vi "practica9.vi"() -> ()   [LabVIEW 2016]
panel:
  in  "file path (use dialog) 2":path
  out "Waveform derecho 2":dbl[](graph)
  out "Waveform izquierdo":dbl[](graph)
  in  "file path (use dialog)":path
  out "Angulo":dbl
  out "Plano de trabajo":picture
  in  "Reset":bool
  in  "stop":bool
  out "Motor Izquierda":dbl(slide) scale=-100.0..100.0
  out "Motor Derecha":dbl(slide) scale=-100.0..100.0
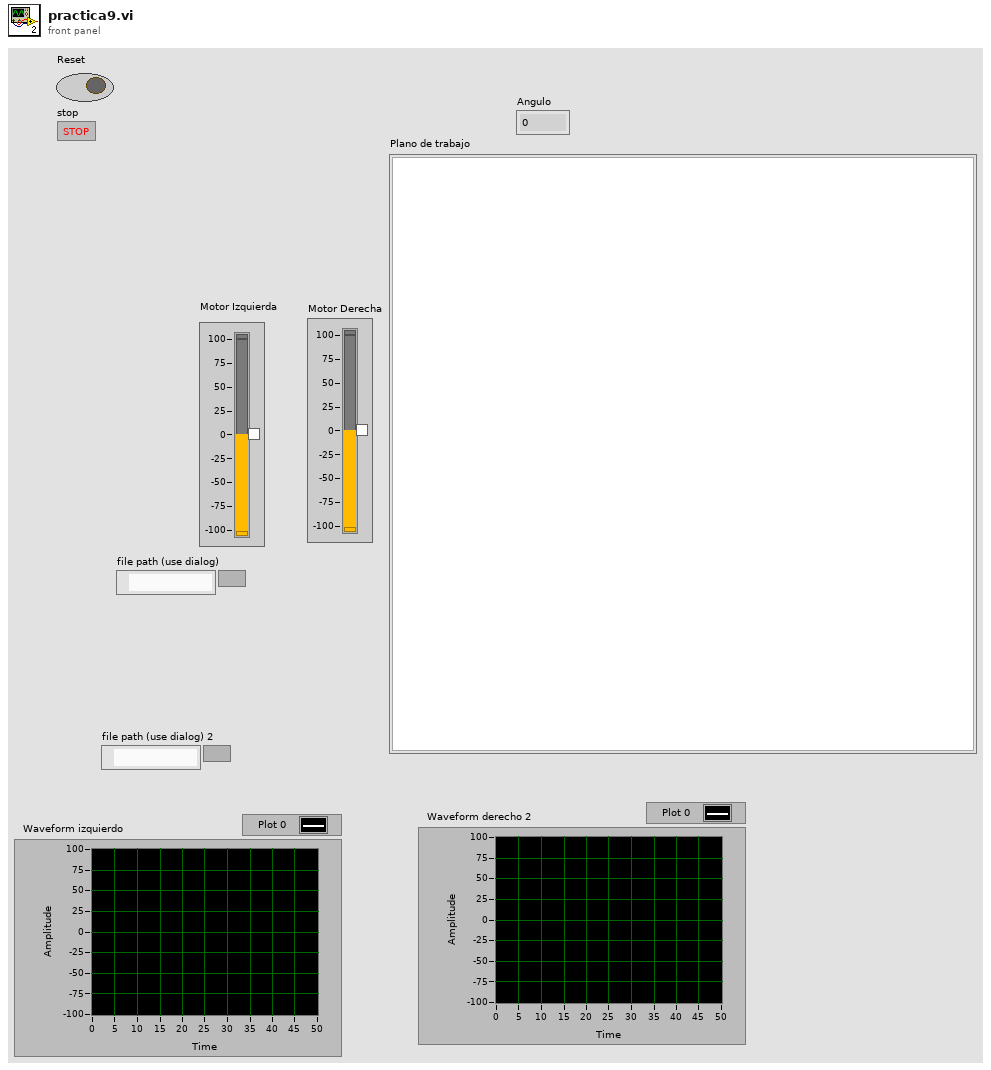
[diagram p1: front panel]
types:
  T1 = enum16{"open", "replace", "create", "open or create", "replace or create", "replace or create with confirmation"}
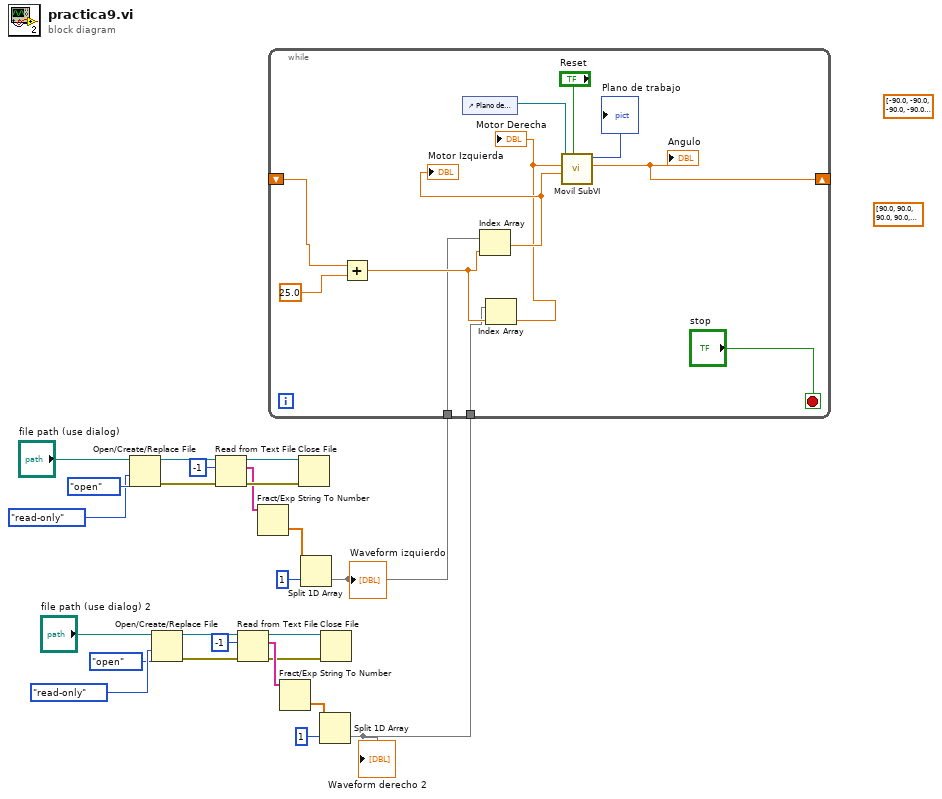
[diagram p0: block diagram]
diagram:
  (unwired) dbl[] [90.0, 90.0, 90.0, 90.0, 90.0, 90.0, 90.0, 90.0, 90.0, 90.0, 90.0, 82.0, 74.0, 66.0, 58.0, 50.0, 50.0, 50.0, 50.0, 50.0, 50.0, 33.3333333333333, 21.4285714285714, 12.5, 5.55555555555556, 0.0, -5.55555555555556, -12.5, -21.4285714285714, -33.3333333333333, -50.0, -50.0, -50.0, -50.0, -50.0, -50.0, -58.0, -66.0, -74.0, -82.0, -90.0, -90.0, -90.0, -90.0, -90.0, -90.0, -90.0, -90.0, -90.0, -90.0, -90.0] ("motor derecha 2")
  (unwired) dbl[] [-90.0, -90.0, -90.0, -90.0, -90.0, -90.0, -90.0, -90.0, -90.0, -90.0, -90.0, -82.0, -74.0, -66.0, -58.0, -50.0, -50.0, -50.0, -50.0, -50.0, -50.0, -33.3333333333333, -21.4285714285714, -12.5, -5.55555555555556, 0.0, 5.55555555555556, 12.5, 21.4285714285714, 33.3333333333333, 50.0, 50.0, 50.0, 50.0, 50.0, 50.0, 58.0, 66.0, 74.0, 82.0, 90.0, 90.0, 90.0, 90.0, 90.0, 90.0, 90.0, 90.0, 90.0, 90.0, 90.0] ("motor izquierda 2")
  n1 = Open/Create/Replace File(file path (use dialog)="file path (use dialog)", operation (0:open)=T1."open", access (0:read/write)=enum16{"read/write", "read-only", "write-only"}."read-only") -> (refnum out=w22:refnum<file>, error out=w20:errorcluster)  [unwired: 3 in, 1 out]
  n2 = Open/Create/Replace File(file path (use dialog)="file path (use dialog) 2", operation (0:open)=T1."open", access (0:read/write)=enum16{"read/write", "read-only", "write-only"}."read-only") -> (refnum out=w5:refnum<file>, error out=w7:errorcluster)  [unwired: 3 in, 1 out]
  n3 = Read from Text File(file (use dialog)=w22, count=-1, error in=w20) -> (refnum out=w23:refnum<file>, text=w16:string[], error out=w21:errorcluster)  [unwired: 1 in, 1 out]
  n4 = Read from Text File(file (use dialog)=w5, count=-1, error in=w7) -> (refnum out=w4:refnum<file>, text=w11:string[], error out=w6:errorcluster)  [unwired: 1 in, 1 out]
  n5 = Fract/Exp String To Number(string=w16) -> (number=w15:dbl[])  [unwired: 3 in, 1 out]
  n6 = Fract/Exp String To Number(string=w11) -> (number=w12:dbl[])  [unwired: 3 in, 1 out]
  n7 = Close File(refnum=w23, error in=w21) -> ()  [unwired: 2 out]
  n8 = Split 1D Array(array=w15, index=1) -> (second subarray=w2:dbl[])  [unwired: 1 out]
  "Waveform izquierdo" <- w2
  n9 = Split 1D Array(array=w12, index=1) -> (second subarray=w1:dbl[])  [unwired: 1 out]
  "Waveform derecho 2" <- w1
  n10 = while {
    shift-right: [w32] -> _
    shift-left: _ -> [w30]
    tunnel: w2 -> [w26]
    tunnel: w1 -> [w25]
    stop <- "stop" stop-if-true
    n11 = Add(x=w30, y=25.0) -> (x+y=w29:dbl)
    n12 = control-ref of="Plano de trabajo"() -> (w35:refnum<vi>)
    n13 = Index Array(array=w26, index=w29) -> (element=w28:dbl)
    "Motor Izquierda" <- w28
    n14 = Index Array(array=w25, index=w29) -> (element=w27:dbl)
    "Motor Derecha" <- w27
    n15 = call "Movil SubVI.vi"("Reset"="Reset", "Motor Izquierda"=w28, "Motor Derecha"=w27, "Ref Plano"=w35) -> ("Angulo"=w32:dbl, "Plano de trabajo"=→"Plano de trabajo":picture)  [unwired: 3 in, 3 out]
    "Angulo" <- w32
  }
  n16 = Close File(refnum=w4, error in=w6) -> ()  [unwired: 2 out]
